vi "USB serial.vi"() -> ()   [LabVIEW 2018]
uses:
  <vilib>/Instr/_visa.llb/VISA Configure Serial Port (Instr).vi
panel:
  out "Milliseconds":dbl format="%.3f"
  in  "MilliSeconsds":dbl(knob) scale=0.0..100.0
  in  "write buffer":string
  out "Serial Settings:Number of Bytes at Serial Port":u32
  out "error out":errorcluster
  in  "E-Stop":bool
  out "read buffer":string
  in  "error in (no error)":errorcluster
  in  "VISA resource name":refnum<visa-resource-name>
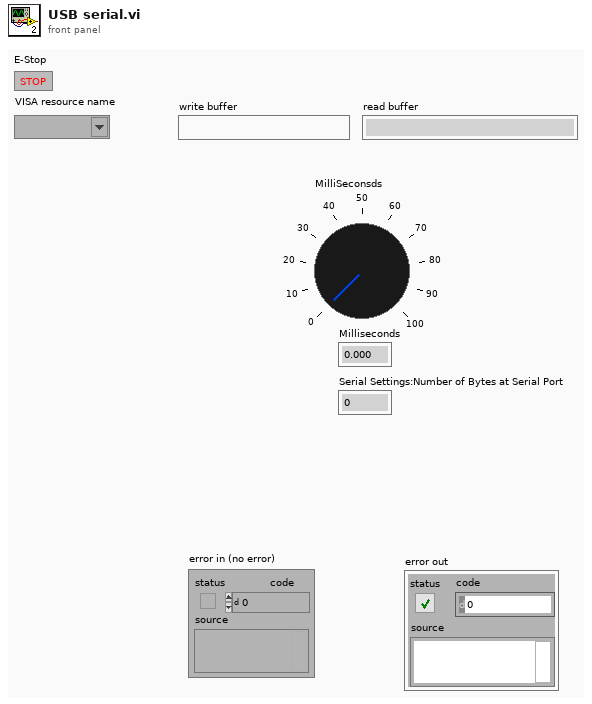
[diagram p1: front panel]
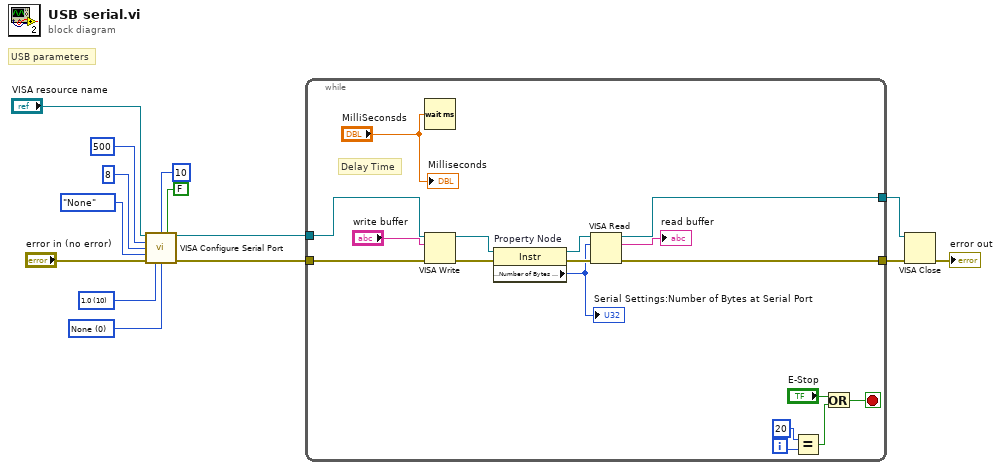
[diagram p0: block diagram]
diagram:
  w6 = u16 0 items=["None", "XON/XOFF", "RTS/CTS", "XON/XOFF & RTS/CTS", "DTR/DSR", "XON/XOFF & DTR/DSR"] ("flow control (0:none)")
  w7 = u16 10 items=["1.0"=10, "1.5"=15, "2.0"=20] ("stop bits (10: 1 bit)")
  # "USB parameters"
  n1 = call-poly "VISA Configure Serial Port"("VISA resource name"="VISA resource name", "termination char\n(0xA = '\\n' = LF)"=u8 10 ("termination char\n(0xA = '\\n' = LF)"), "Enable Termination\nChar (T)"=FALSE ("Enable Termination\nChar (T)"), "baud rate (9600)"=u32 500, "data bits (8)"=u16 8, "parity (0:none)"=enum16{"None", "Odd", "Even", "Mark", "Space"}."None", "error in (no error)"="error in (no error)", "stop bits (10: 1 bit)"=w7, "flow control (0:none)"=w6) -> ("VISA resource name out"=w8:refnum<visa-resource-name>, "error out"=w9:errorcluster)  [unwired: 5 in]
  n2 = while {
    tunnel: w9 -> [w31]
    tunnel: w8 -> [w30]
    tunnel: [w21] -> w5
    tunnel: [w20] -> w4
    i -> [w18]
    stop <- w16 stop-if-true
    # "Delay Time"
    n3 = Wait (ms)(milliseconds to wait="MilliSeconsds") -> ()  [unwired: 1 out]
    n4 = VISA Write(VISA resource name=w30, write buffer="write buffer", error in (no error)=w31) -> (VISA resource name out=w29:refnum<visa-resource-name>, error out=w28:errorcluster)  [unwired: 1 out]
    n5 = property on="Property Node" class="Instr"(reference=w29, error in=w28) -> (reference out=w26:refnum<visa-resource-name>, error out=w27:errorcluster, "Serial Settings:Number of Bytes at Serial Port"=w25:u32)
    "Serial Settings:Number of Bytes at Serial Port" <- w25
    n6 = VISA Read(VISA resource name=w26, byte count=w25, error in (no error)=w27) -> (VISA resource name out=w21:refnum<visa-resource-name>, read buffer=→"read buffer":string, error out=w20:errorcluster)  [unwired: 1 out]
    n7 = Equal?(x=20, y=w18) -> (x = y?=w15:bool)
    n8 = Or(x="E-Stop", y=w15) -> (x .or. y?=w16:bool)
    "Milliseconds" <- "MilliSeconsds"
  }
  n9 = VISA Close(VISA resource name=w5, error in (no error)=w4) -> (error out=→"error out":errorcluster)
